vi "FFT_wohost.vi"() -> ()   [LabVIEW 2020]
uses:
  <vilib>/rvi/Analysis/measure/FFT/simModelSupport/niFPGA FFT Outside SCTL Sim Properties.ctl
  <vilib>/rvi/Analysis/measure/FFT/simModelSupport/niFPGA FFT Sim Types.ctl
  <vilib>/rvi/Analysis/measure/FFT/simModelSupport/niFpgaFFTSimArithmeticProperties.ctl
  <vilib>/rvi/Analysis/measure/FFT/simModelSupport/niFpgaFFTSimDfxp.ctl
  <vilib>/fxp/LVFixedPointQuantizationPolicyTypeDef.ctl
  <vilib>/rvi/Emulation/niFpgaGetClockAttributes.vi
  <vilib>/rvi/Emulation/niFpgaSctlEmulationGetInTimedLoop.vi
  <vilib>/rvi/Emulation/niFpgaEmulationReportErrorSimple.vi
  <vilib>/rvi/interface/RandomDataEmulation/niFpgaRandomDataHandleErrors.vi
  <vilib>/rvi/Analysis/measure/FFT/simModelSupport/niFpgaFFTSimModelOutsideSCTLCore.vi
  <vilib>/rvi/Emulation/niFpgaCriticalErrorInLSC.vi
  <vilib>/rvi/DataTransferAndStorage/Container/XNode/niFpgaContainer.xnode
  <vilib>/rvi/interface/RandomDataEmulation/nirviRandomDataFpgaReadWriteTemplate.vi
  <vilib>/rvi/Analysis/measure/FFT/XNode/niFpgaFFT.xnode
panel:
  out "x-y (microsecond)":u32
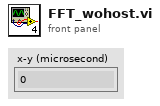
[diagram p1: front panel]
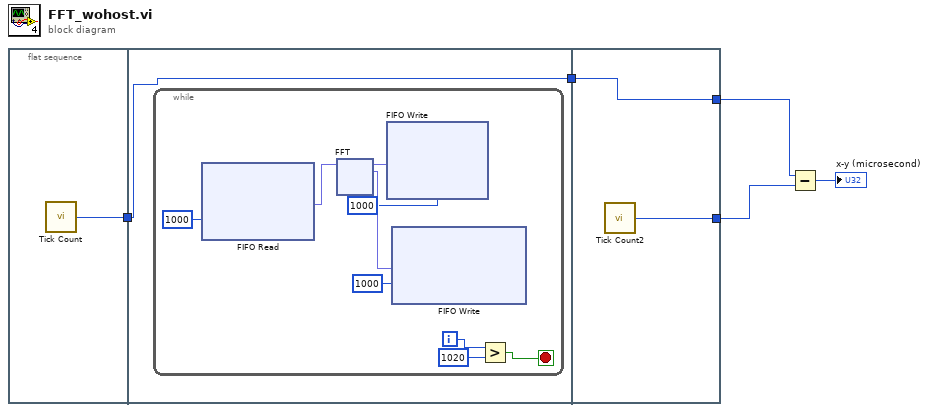
[diagram p0: block diagram]
diagram:
  n1 = flat-sequence {
    tunnel: [w6] -> w5
    tunnel: [w7] -> w4
    tunnel: w5 -> [w7]
    tunnel: [w38] -> w3
    tunnel: w4 -> [w38]
    tunnel: [w37] -> w2
    frame #0 {
      n2 = call "Tick Count"() -> ("Tick Count(uSec)"=w6:u32)
    }
    frame #1 {
      n3 = while {
        i -> [w10]
        stop <- w8 stop-if-true
        n4 = xnode ("FIFO Read")("Timeout"=1000) -> ("Element"=w16:fxp<+/-,32,16>)  [unwired: 1 in, 2 out]
        n5 = xnode "FFT"("real data in"=w16) -> ("real data out"=w15:fxp<+/-,31,23>, "imaginary data out"=w14:fxp<+/-,31,23>)  [unwired: 2 in, 2 out]
        n6 = xnode ("FIFO Write")("Element"=w15, "Timeout"=1000) -> ()  [unwired: 1 in, 2 out]
        n7 = xnode ("FIFO Write")("Element"=w14, "Timeout"=1000) -> ()  [unwired: 1 in, 2 out]
        n8 = Greater?(x=w10, y=1020) -> (0:w8:bool)
      }
    }
    frame #2 {
      n9 = call "Tick Count2"() -> ("Tick Count(uSec)"=w37:u32)
    }
  }
  n10 = Subtract(x=w3, y=w2) -> (x-y=→"x-y (microsecond)":u32)
